vi "HC MFR sw 1.vi"(9 "HC Conc %":dbl, 10 "C_HC":dbl, 11 "Flow rate":dbl) -> (3 "HC MFR":dbl)   [LabVIEW 2014]
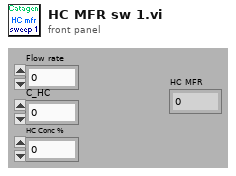
[diagram p1: front panel]
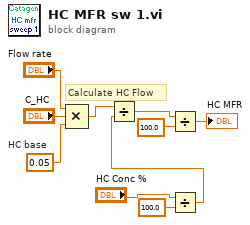
[diagram p0: block diagram]
diagram:
  w6 = 0.05  # HC base
  # "Calculate HC Flow"
  n1 = Compound Arithmetic op=MULTIPLY("Flow rate", "C_HC", w6) -> (w3:dbl)
  n2 = Divide(x="HC Conc %", y=100.0) -> (x/y=w2:dbl)
  n3 = Divide(x=w3, y=w2) -> (x/y=w1:dbl)
  n4 = Divide(x=w1, y=100.0) -> (x/y=→"HC MFR":dbl)
